vi "Add DUT SIM Slot.vi"(8 "error in (no error)":errorcluster, 9 "SIM Profile (\"SIM1\")":string="SIM1", 10 "DUT (\"DUT1\")":string="DUT1", 11 "VISA resource name":refnum<visa-resource-name>) -> (0 "error out":errorcluster, 3 "VISA resource name out":refnum<visa-resource-name>)   [LabVIEW 2020, in "Rohde&Schwarz CMXP Base.lvlib"]
doc: "Adds a SIM slot with the assigned SIM profile name to the inactive DUT with the specified name.\n\nAssign a unique name to each named object within the test environment. Assigning an already used name can be rejected with an error message, even if the other object has not the same type as the new object.\n\nAttribute:\n-\n\nRemote-control command:\nCREate:DUT:PROFile:SIMSlot"
uses:
  <instrlib>/Rohde&Schwarz CMXP Base/Rohde&Schwarz CMXP Base.lvlib
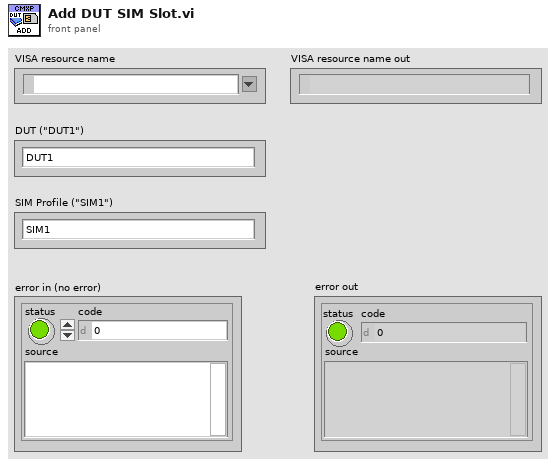
[diagram p1: front panel]
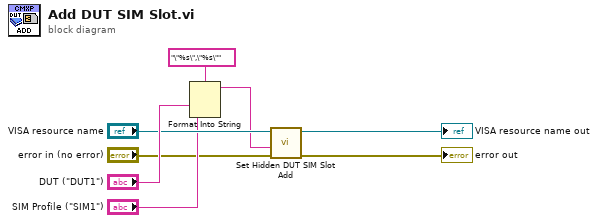
[diagram p0: block diagram]
diagram:
  n1 = Format Into String(format string="\"%s\",\"%s\"", "DUT (\"DUT1\")", "SIM Profile (\"SIM1\")") -> (resulting string=w1:string)  [unwired: 2 in, 1 out]
  n2 = call "Set Hidden DUT SIM Slot Add"("error in (no error)"="error in (no error)", "Hidden DUT SIM Slot Add ()"=w1, "instrument handle"="VISA resource name") -> ("error out"=→"error out":errorcluster, "instrument handle out"=→"VISA resource name out":refnum<visa-resource-name>)  [unwired: 7 in]
